vi "send_burleighJump-v02.vi"(0 "daq_ao 2":tag="Dev1/ao1", 1 "daq_ai":tag="Dev1/ai0:1", 2 "Jump Polarity":bool, 5 "Duration (s)":dbl, 7 "Sample Freq (Hz)":dbl min=0.0 max=40000.0, 9 "Phase":dbl, 11 "Duty Cycle":dbl, 12 "Jump Filter Freq (Hz)":dbl=20.0 min=0.0 max=40000.0, 13 "Number of Replicates":i16=1 min=1 max=10, 14 "error in":errorcluster) -> (4 "output cluster":T1={"daq_ao 2"="", "Duration (s)"=0.0, "Sample Freq (Hz)"=0.0, "Phase"=0.0, "Duty Cycle"=0.0, "Jump Filter Freq (Hz)"=0.0, "Number of Replicates"=1} {"Number of Replicates" min=1 max=10}, 6 "output waveform":waveform(dbl)(graph), 8 "protocol response":waveform(dbl)[](graph) caption="jumptestMonitor", 10 "error out":errorcluster)   [LabVIEW 2019]
uses:
  <vilib>/Analysis/3filter.llb/Filter Passband Type.ctl
  <vilib>/Analysis/3filter.llb/Bessel Filter (DBL).vi
  <vilib>/measure/NI_MABase.lvlib
  <vilib>/Analysis/NI_AALBase.lvlib
panel:
  # "Low"
  # "High"
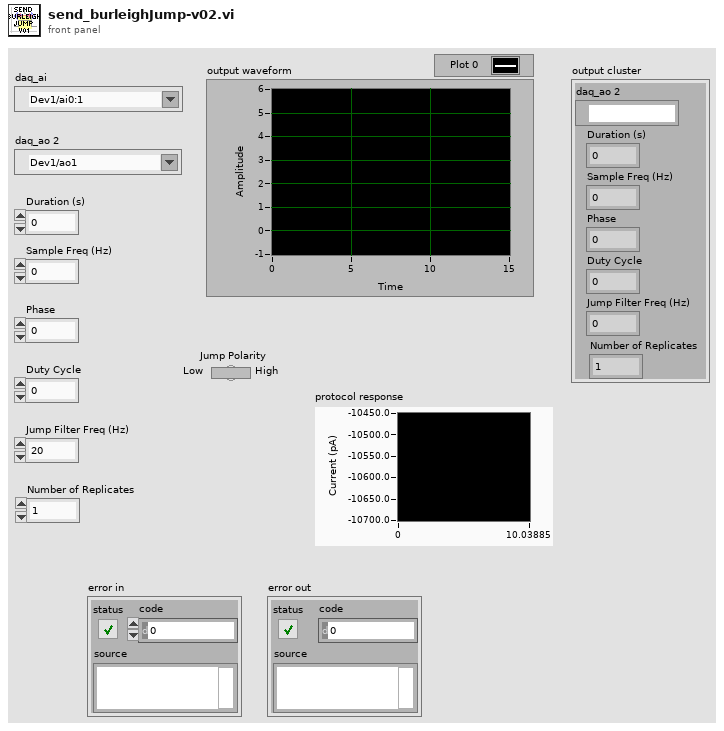
[diagram p1: front panel]
types:
  T1 = cluster{"daq_ao 2":tag, "Duration (s)":dbl, "Sample Freq (Hz)":dbl, "Phase":dbl, "Duty Cycle":dbl, "Jump Filter Freq (Hz)":dbl, "Number of Replicates":i16}
  T2 = typedef "NI_AALBase.lvlib/Filter Passband Type.ctl" = enum32{"Lowpass", "Highpass", "Bandpass", "Bandstop"}
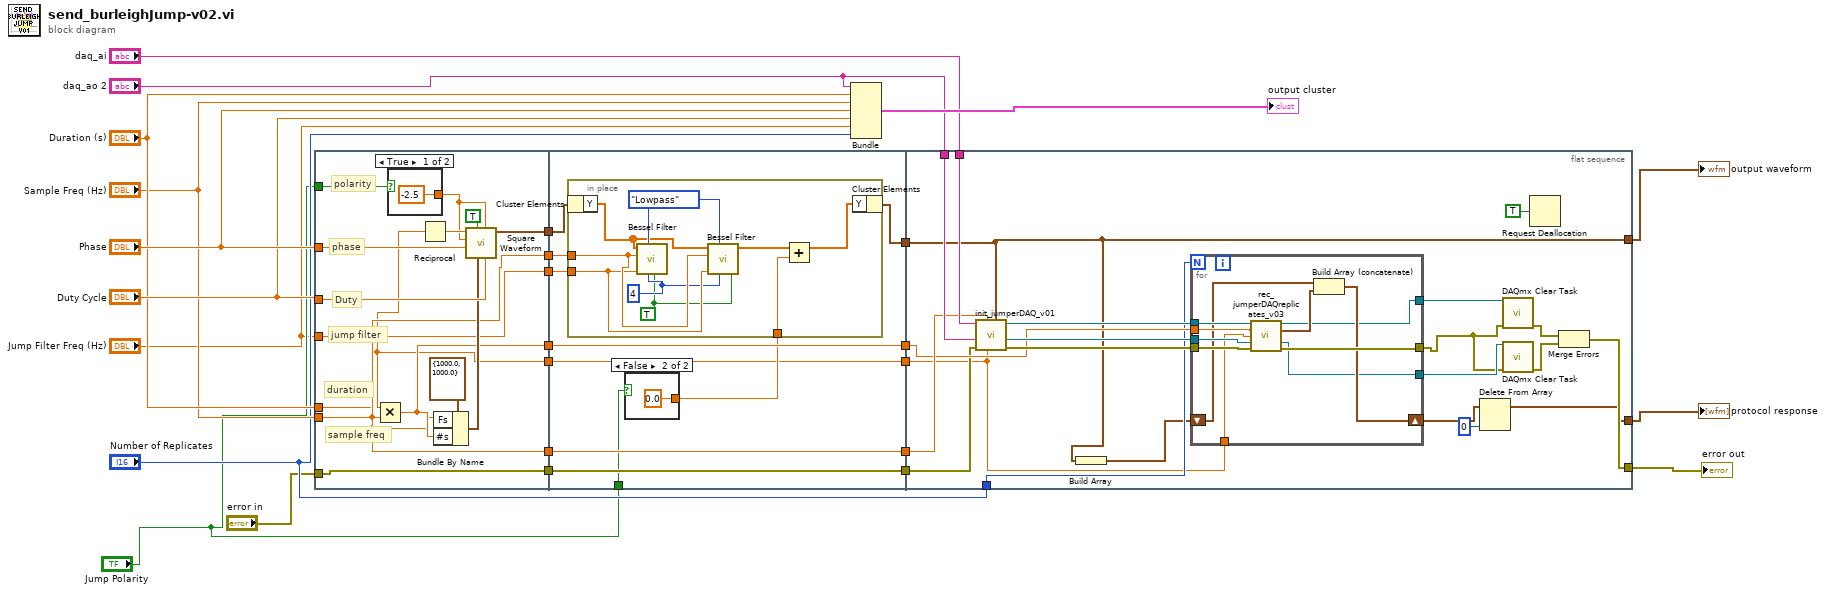
[diagram p0: block diagram]
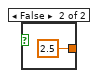
[diagram p2: hidden frame]
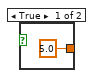
[diagram p3: hidden frame]
diagram:
  n1 = flat-sequence {
    tunnel: "Phase" -> [w40]
    tunnel: "Duty Cycle" -> [w39]
    tunnel: "Duration (s)" -> [w27]
    tunnel: "Jump Filter Freq (Hz)" -> [w34]
    tunnel: "Sample Freq (Hz)" -> [w33]
    tunnel: [w35] -> w17
    tunnel: [w33] -> w14
    tunnel: [w34] -> w12
    tunnel: [w33] -> w11
    tunnel: [w32] -> w10
    tunnel: "error in" -> [w30]
    tunnel: [w30] -> w6
    tunnel: "Jump Polarity" -> [w29]
    tunnel: [w27] -> w2
    tunnel: w17 -> [w52]
    tunnel: [w52] -> w16
    tunnel: [w44] -> w15
    tunnel: w14 -> [w51]
    tunnel: [w51] -> w13
    tunnel: w12 -> [w45]
    tunnel: w11 -> [w46]
    tunnel: w10 -> [w43]
    tunnel: [w50] -> w7
    tunnel: w6 -> [w50]
    tunnel: "Jump Polarity" -> [w48]
    tunnel: w2 -> [w47]
    tunnel: [w47] -> w1
    tunnel: [w64] -> w22
    tunnel: w16 -> [w79]
    tunnel: w15 -> [w64]
    tunnel: "daq_ai" -> [w82]
    tunnel: "daq_ao 2" -> [w81]
    tunnel: w13 -> [w80]
    tunnel: [w68] -> w19
    tunnel: "Number of Replicates" -> [w78]
    tunnel: [w72] -> w5
    tunnel: w7 -> [w77]
    tunnel: w1 -> [w66]
    frame #0 {
      # "sample freq"
      # "duration"
      # "jump filter"
      # "Duty"
      # "phase"
      # "polarity"
      n2 = Multiply(x=w27, y=w33) -> (x*y=w35:dbl)
      n3 = case shown="True" w29 {
        tunnel: [-2.5 ("Amplitude") 2.5 ("Amplitude")] -> w28
        frame True {
        }
        frame False {
        }
      }
      n4 = Reciprocal(x=w27) -> (1/x=w31:dbl)
      n5 = Bundle By Name(cluster=cluster{"Fs":dbl, "#s":dbl} {"Fs"=1000.0, "#s"=1000.0} ("sampling info"), "Fs"=w33, "#s"=w35) -> (w36:cluster{"Fs":dbl, "#s":dbl})
      n6 = call <vilib>:"Square Waveform.vi"("duty cycle (%)"=w39, "offset"=w28, "sampling info"=w36, "reset signal"=TRUE, "phase"=w40, "amplitude"=w28, "frequency"=w31) -> ("signal out"=w32:waveform(dbl))  [unwired: 3 in, 1 out]
    }
    frame #1 {
      n7 = case shown="False" w48 {
        tunnel: [5.0 ("Amplitude") 0.0 ("Amplitude")] -> w49
        frame True {
        }
        frame False {
        }
      }
      n8 = in-place {
        in-place-border: w49 -> [w61]
        in-place-border: w46 -> [w60]
        in-place-border: w45 -> [w59]
        w57 = TRUE ("init/cont (init:F)")
        w58 = 4 ("order")
        w56 = Filter_Passband_Type."Lowpass" ("filter type")
        n9 = in-place-cluster #1(w43) -> ("Y"=w53:dbl[])
        n10 = call-poly <vilib>:"Bessel Filter.vi"("init/cont (init:F)"=w57, "order"=w58, "filter type"=w56, "low cutoff freq: fl"=w59, "sampling freq: fs"=w60, "X"=w53) -> ()  [unwired: 2 in, 2 out]
        n11 = call-poly <vilib>:"Bessel Filter.vi"("init/cont (init:F)"=w57, "order"=w58, "filter type"=w56, "low cutoff freq: fl"=w59, "sampling freq: fs"=w60, "X"=w53) -> ("Filtered X"=w55:dbl[])  [unwired: 2 in, 1 out]
        n12 = Add(x=w55, y=w61) -> (x+y=w54:dbl[])
        n13 = in-place-cluster #1("Y"=w54) -> (w44:waveform(dbl))
      }
    }
    frame #2 {
      n14 = call "init_jumperDAQ_v01.vi"("protocol waveform"=w64, "Duration (s)"=w66, "Sample Freq (Hz)"=w80, "AO error in"=w77, "AO physical channels"=w81, "AI Physical Channel"=w82) -> ("AO error out"=w85:errorcluster, "AO task out"=w84:refnum<k21>, "AI task out"=w83:refnum<k21>)  [unwired: 1 in, 2 out]
      n15 = Build Array(w64) -> (w70:waveform(dbl)[])
      n16 = for {
        N: w78 -> [_]
        tunnel: w85 -> [w96]
        tunnel: w84 -> [w95]
        tunnel: w83 -> [w94]
        tunnel: w79 -> [w92]
        shift-right: [w90] -> w69
        shift-left: w70 -> [w89]
        tunnel: [w93] -> w74
        tunnel: [w88] -> w76
        tunnel: [w87] -> w75
        tunnel: w66 -> [w86]
        n17 = call "rec_jumperDAQreplicates_v03.vi"("AI task in"=w94, "number of samples"=w92, "Duration (s)"=w86, "AO task in"=w95, "error in"=w96) -> ("AI task out"=w87:refnum<k21>, "data out (pA or mV)"=w91:waveform(dbl), "AO task out"=w88:refnum<k21>, "error out"=w93:errorcluster)  [unwired: 7 in]
        n18 = Build Array (concatenate)(w89, w91) -> (w90:waveform(dbl)[])
      }
      n19 = Delete From Array(array=w69, index=0) -> (array with subset deleted=w68:waveform(dbl)[])  [unwired: 1 in, 1 out]
      n20 = call <vilib>:"DAQmx Clear Task.vi"("task in"=w75, "error in"=w74) -> ("error out"=w71:errorcluster)  [unwired: 13 in]
      n21 = call <vilib>:"DAQmx Clear Task.vi"("task in"=w76, "error in"=w74) -> ("error out"=w73:errorcluster)  [unwired: 13 in]
      n22 = Request Deallocation(TRUE ("flag")) -> ()
      n23 = Merge Errors(w71, w73) -> (w72:errorcluster)
    }
  }
  n24 = Bundle("daq_ao 2"="daq_ao 2", "Duration (s)"="Duration (s)", "Sample Freq (Hz)"="Sample Freq (Hz)", "Phase"="Phase", "Duty Cycle"="Duty Cycle", "Jump Filter Freq (Hz)"="Jump Filter Freq (Hz)", "Number of Replicates"="Number of Replicates") -> (→"output cluster":T1)  [unwired: 1 in]
  "protocol response" <- w19
  "output waveform" <- w22
  "error out" <- w5
